vi "Temperature controller differential.vi"() -> ()   [LabVIEW 2011]
uses:
  <vilib>/Utility/error.llb/DialogType.ctl
  <vilib>/DAQmx/write.llb/DAQmx Write (Analog DBL 1Chan 1Samp).vi
  <vilib>/DAQmx/read.llb/DAQmx Read (Analog 2D DBL NChan NSamp).vi
  <vilib>/DAQmx/miscellaneous.llb/DAQmx Fill In Error Info.vi
  <vilib>/Analysis/NI_AALBase.lvlib
  <vilib>/addons/control/pid/NI_PID_autopid.lvlib
panel:
  in  "Heater master power switch 2":refnum<k21>="Dev2_ao1"
  in  "temp sensor channels":tag="Dev3/ai2:3"
  in  "PID gains":T1={"proportional gain (Kc)"=10.0, "integral time (Ti, min)"=0.0, "derivative time (Td, min)"=0.0} {"derivative time (Td, min)" format="%.3f"; "integral time (Ti, min)" format="%.3f"; "proportional gain (Kc)" format="%.3f"}
  in  "reinitialize? (F)":bool
  out "Heater output":dbl=0.7 format="%.2f"
  out "PID gains out":T1={"proportional gain (Kc)"=10.0, "integral time (Ti, min)"=0.0, "derivative time (Td, min)"=0.0} {"derivative time (Td, min)" format="%.3f"; "integral time (Ti, min)" format="%.3f"; "proportional gain (Kc)" format="%.3f"}
  out "tuning completed?":bool
  in  "autotune? (F)":bool
  in  "Temperature\nsetpoint":dbl=20.0 format="%.2f"
  in  "Heater master power switch":refnum<k21>="Dev2_ao0"
  in  "heater channel":refnum<k21>="Dev3_ao1"
  in  "stop":bool
  out "Waveform Chart":T2(graph)={"mean"=23.930114733929784, "mean"=22.350166073494023, "Temperature\nsetpoint"=20.0, "output"=0.7}
  in  "error in":errorcluster
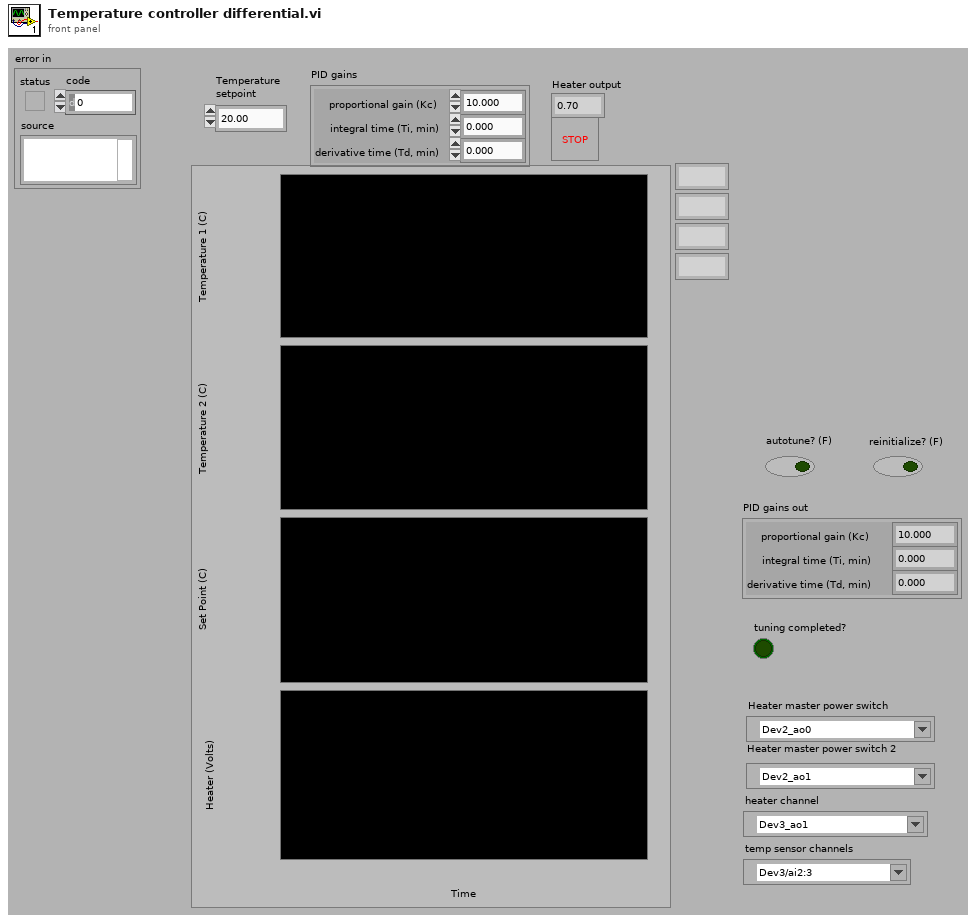
[diagram p1: front panel]
types:
  T1 = cluster{"proportional gain (Kc)":dbl, "integral time (Ti, min)":dbl, "derivative time (Td, min)":dbl}
  T2 = cluster{"mean":dbl, "mean":dbl, "Temperature\nsetpoint":dbl, "output":dbl}
  T3 = enum16{"open", "replace", "create", "open or create", "replace or create", "replace or create with confirmation"}
  T4 = typedef "DialogType.ctl" = u16
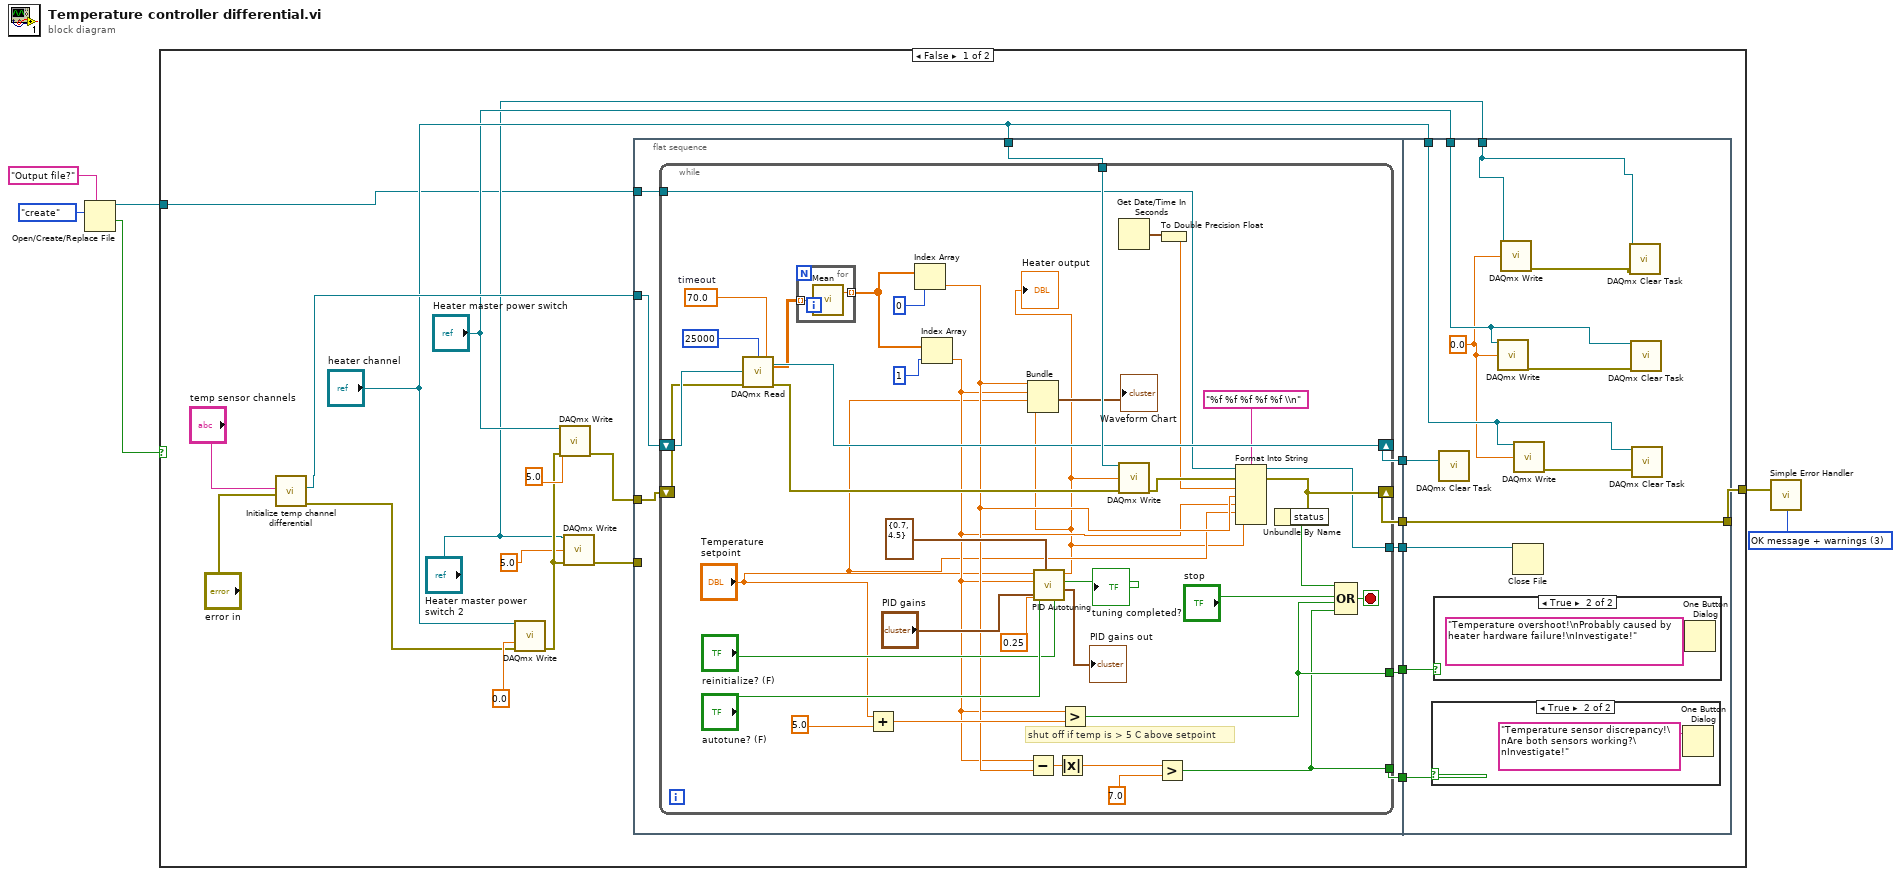
[diagram p0: block diagram]
diagram:
  w5 = T4 3 items=["no dialog", "OK message", "continue or stop message", "OK message + warnings", "continue/stop + warnings"] ("type of dialog (OK msg:1)")
  n1 = Open/Create/Replace File(prompt="Output file?", operation (0:open)=T3."create") -> (refnum out=w3:refnum<file>, cancelled=w1:bool)  [unwired: 4 in, 1 out]
  n2 = case shown="False" w1 {
    tunnel: [w19 _] -> w6
    tunnel: w3 -> [w7 _]
    frame False {
      n3 = call "Initialize temp channel differential.vi"("error in"="error in", "Physical channel"="temp sensor channels") -> ("error out"=w18:errorcluster, "task out"=w14:refnum<k21>)  [unwired: 6 in]
      n4 = call-poly <vilib>:"DAQmx Write.vi"("task/channels in"="heater channel", "data"=0.0, "error in"=w18) -> ("error out"=w11:errorcluster)  [unwired: 1 in, 11 out]
      n5 = call-poly <vilib>:"DAQmx Write.vi"("task/channels in"="Heater master power switch", "data"=5.0, "error in"=w11) -> ("error out"=w15:errorcluster)  [unwired: 1 in, 11 out]
      n6 = call-poly <vilib>:"DAQmx Write.vi"("task/channels in"="Heater master power switch 2", "data"=5.0, "error in"=w11) -> ("error out"=w8:errorcluster)  [unwired: 1 in, 11 out]
      n7 = flat-sequence {
        tunnel: w14 -> [w35]
        tunnel: "heater channel" -> [w33]
        tunnel: [w34] -> w26
        tunnel: [w32] -> w25
        tunnel: [w31] -> w24
        tunnel: [w30] -> w23
        tunnel: w15 -> [w29]
        tunnel: w8 -> [_]
        tunnel: w7 -> [w28]
        tunnel: [w27] -> w22
        tunnel: [w89] -> w19
        tunnel: w26 -> [w88]
        tunnel: w25 -> [w89]
        tunnel: "heater channel" -> [w82]
        tunnel: "Heater master power switch" -> [w87]
        tunnel: w24 -> [w84]
        tunnel: w23 -> [w83]
        tunnel: "Heater master power switch 2" -> [w80]
        tunnel: w22 -> [w78]
        frame #0 {
          n8 = while {
            shift-right: [w45] -> w32
            shift-left: w29 -> [w63]
            shift-right: [w61] -> w34
            shift-left: w35 -> [w64]
            tunnel: w33 -> [w72]
            tunnel: [w50] -> w31
            tunnel: [w49] -> w30
            tunnel: w28 -> [w44]
            tunnel: [w43] -> w27
            stop <- w67 stop-if-true
            w54 = 70.0  # timeout
            # "shut off if temp is > 5 C above setpoint"
            n9 = call-poly <vilib>:"DAQmx Read.vi"("task/channels in"=w64, "number of samples per channel"=25000, "timeout"=w54, "error in"=w63) -> ("task out"=w61:refnum<k21>, "data"=w47:dbl[][], "error out"=w62:errorcluster)  [unwired: 9 out]
            n10 = for {
              tunnel: [w77] -> w58 mode=indexing
              tunnel: w47 -> [w76] mode=indexing
              n11 = call <vilib>:"Mean.vi"("X"=w76) -> ("mean"=w77:dbl)  [unwired: 1 out]
            }
            n12 = Add(x="Temperature\nsetpoint", y=5.0) -> (x+y=w71:dbl)
            n13 = Index Array(array=w58, index=0) -> (element=w41:dbl)
            n14 = Index Array(array=w58, index=1) -> (element=w40:dbl)
            n15 = Subtract(x=w40, y=w41) -> (x-y=w57:dbl)
            n16 = call <vilib>:"PID Autotuning.vi"("autotune? (F)"="autotune? (F)", "reinitialize? (F)"="reinitialize? (F)", "output range"=cluster{"output high":dbl, "output low":dbl} {"output high"=0.7, "output low"=4.5}, "dt (s)"=0.25, "PID gains"="PID gains", "process variable"=w40, "setpoint"="Temperature\nsetpoint") -> ("PID gains out"=→"PID gains out":T1, "tuning completed?"=→"tuning completed?":bool, "output"=w38:dbl)  [unwired: 1 in, 1 out]
            "Heater output" <- w38
            n17 = Bundle("mean"=w41, "mean"=w40, "Temperature\nsetpoint"="Temperature\nsetpoint", "output"=w38) -> (→"Waveform Chart":T2)  [unwired: 1 out]
            n18 = Absolute Value(x=w57) -> (abs(x)=w55:dbl)
            n19 = Greater?(x=w40, y=w71) -> (0:w50:bool)
            n20 = Get Date/Time In Seconds() -> (seconds since 1Jan1904=w37:timestamp)
            n21 = call-poly <vilib>:"DAQmx Write.vi"("task/channels in"=w72, "data"=w38, "error in"=w62) -> ("error out"=w46:errorcluster)  [unwired: 1 in, 11 out]
            n22 = Greater?(x=w55, y=7.0) -> (0:w49:bool)
            n23 = To Double Precision Float(number=w37) -> (double precision float=w36:dbl)
            n24 = Format Into String(format string="%f %f %f %f %f \\n", initial string=w44, error in=w46, w36, w41, w40, "Temperature\nsetpoint", w38) -> (resulting string=w43:refnum<file>, error out=w45:errorcluster)
            n25 = Unbundle By Name(w45) -> ("status"=w69:bool)
            n26 = Compound Arithmetic op=OR(w69, "stop", w50, w49) -> (w67:bool)
          }
        }
        frame #1 {
          w79 = 0.0 ("data")
          n27 = case shown="True" w83 {
            frame False {
            }
            frame True {
              n28 = One Button Dialog(message="Temperature sensor discrepancy!\nAre both sensors working?\nInvestigate!") -> ()  [unwired: 2 out]
            }
          }
          n29 = case shown="True" w84 {
            frame False {
            }
            frame True {
              n30 = One Button Dialog(message="Temperature overshoot!\nProbably caused by heater hardware failure!\nInvestigate!") -> ()  [unwired: 2 out]
            }
          }
          n31 = call <vilib>:"DAQmx Clear Task.vi"("task in"=w88) -> ()  [unwired: 1 in, 14 out]
          n32 = call-poly <vilib>:"DAQmx Write.vi"("task/channels in"=w87, "data"=w79) -> ("error out"=w86:errorcluster)  [unwired: 3 in, 10 out]
          n33 = call-poly <vilib>:"DAQmx Write.vi"("task/channels in"=w80, "data"=w79) -> ("error out"=w81:errorcluster)  [unwired: 3 in, 10 out]
          n34 = Close File(refnum=w78) -> ()  [unwired: 1 in, 2 out]
          n35 = call-poly <vilib>:"DAQmx Write.vi"("task/channels in"=w82, "data"=w79) -> ("error out"=w85:errorcluster)  [unwired: 2 in, 11 out]
          n36 = call <vilib>:"DAQmx Clear Task.vi"("task in"=w80, "error in"=w81) -> ()  [unwired: 14 out]
          n37 = call <vilib>:"DAQmx Clear Task.vi"("task in"=w87, "error in"=w86) -> ()  [unwired: 14 out]
          n38 = call <vilib>:"DAQmx Clear Task.vi"("task in"=w82, "error in"=w85) -> ()  [unwired: 14 out]
        }
      }
    }
    frame True {
    }
  }
  n39 = call <vilib>:"Simple Error Handler.vi"("type of dialog (OK msg:1)"=w5, "error in (no error)"=w6) -> ()  [unwired: 8 out]
